vi "test spiral scan.vi"() -> ()   [LabVIEW 2010]
uses:
  scan_specification_tagResonant.ctl
panel:
  out "Waveform Chart":i16[](graph)
  out "scan pattern":cluster{i16[], i16[]}[](graph)
  out "scan specification out":T1
  out "rev scan pattern":cluster{i16[], i16[]}(graph)
  out "fwd scan pattern":cluster{i16[], i16[]}(graph)
  in  "maximum frequency":dbl=3000.0
  in  "scan specification":T1={"z resolution (pixels)"=30, "iterations per pixel"=5, "iterations per z-scan (=zres*iterperpixel)"=150, "x resolution (pixels)"=80, "y resolution (pixels)"=80, "number of z-lines per volume"=0, "number of repetitions (volumes)"=0, "Pockels cell voltage (bits)"=0, "Vx center (bits)"=0, "Vy center (bits)"=0, "Vx amplitude (bits)"=1000, "Vy amplitude (bits)"=1000, "lines to delay between scan start and output"=0, "LSB has acquire control"=FALSE}
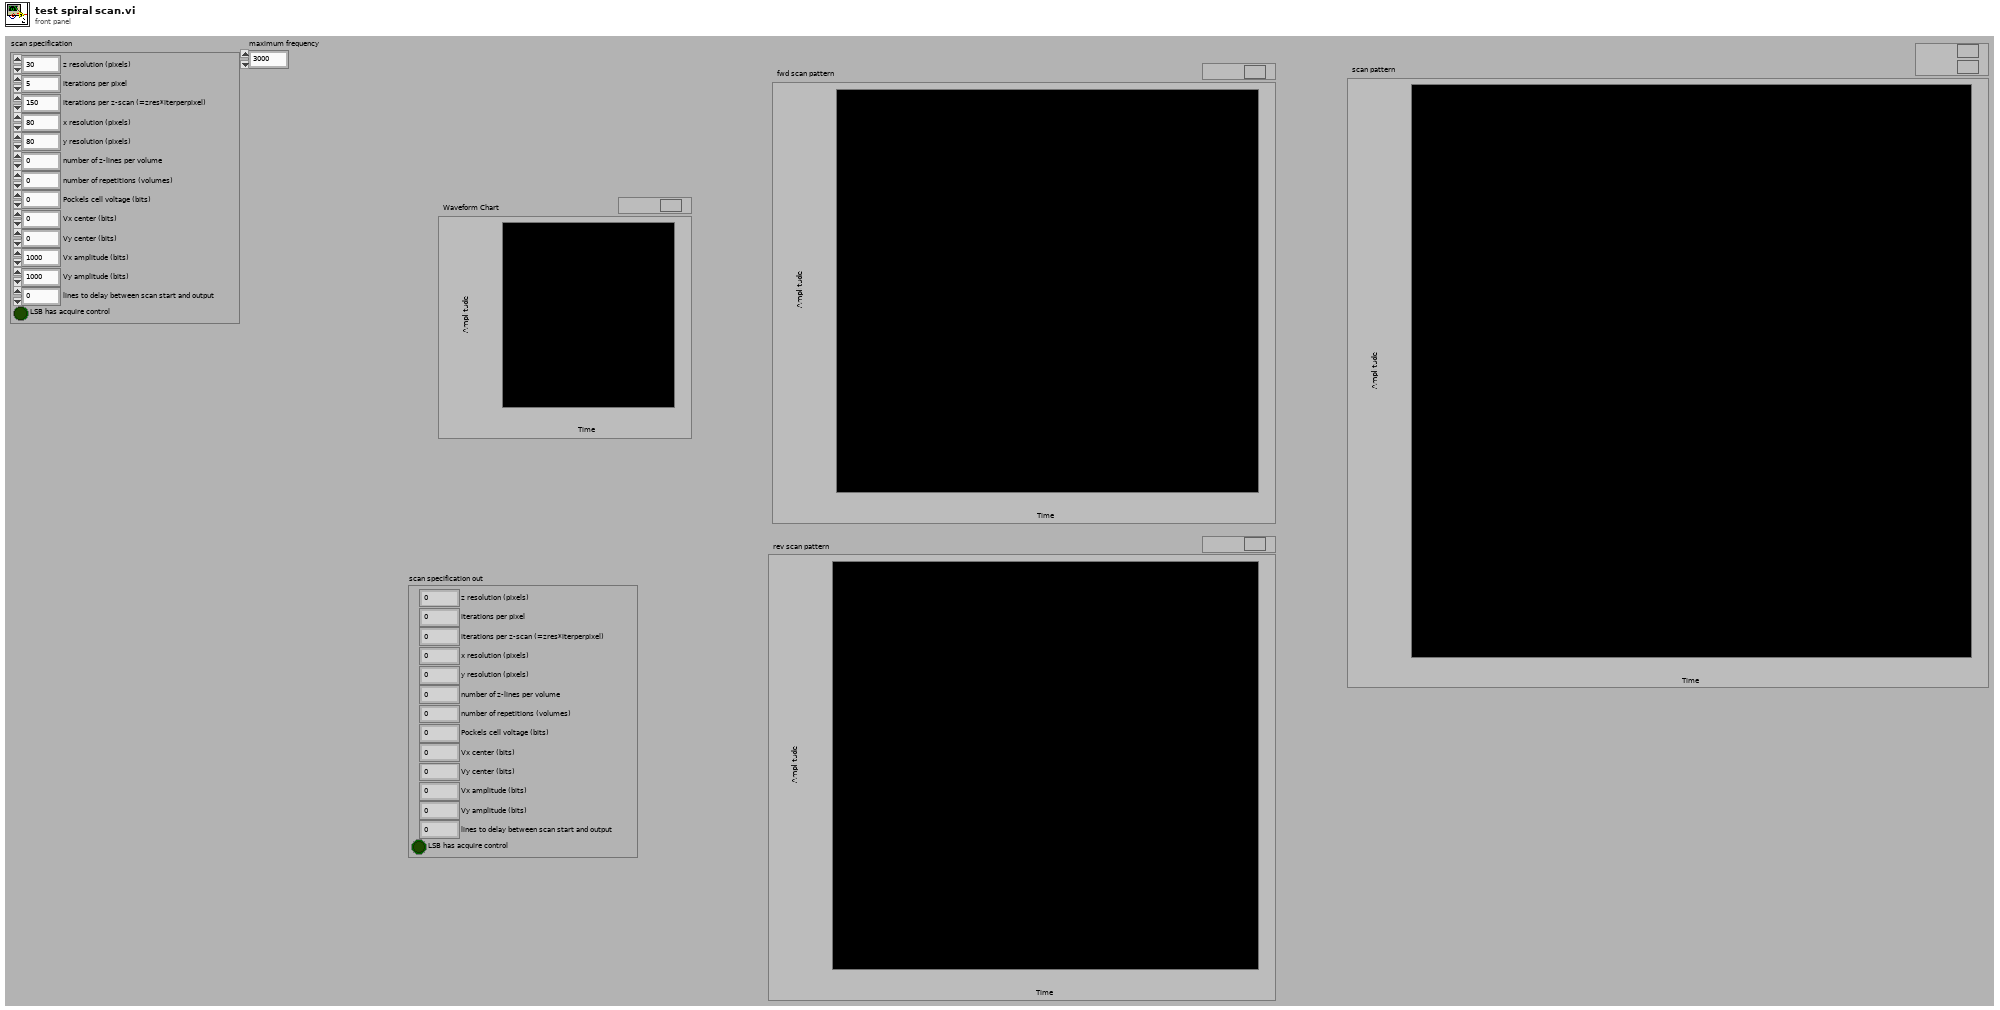
[diagram p1: front panel]
types:
  T1 = typedef "scan_specification_tagResonant.ctl" = cluster{"z resolution (pixels)":u16, "iterations per pixel":u16, "iterations per z-scan (=zres*iterperpixel)":u16, "x resolution (pixels)":u16, "y resolution (pixels)":u16, "number of z-lines per volume":u16, "number of repetitions (volumes)":i32, "Pockels cell voltage (bits)":i16, "Vx center (bits)":i16, "Vy center (bits)":i16, "Vx amplitude (bits)":i16, "Vy amplitude (bits)":i16, "lines to delay between scan start and output":u16, "LSB has acquire control":bool}
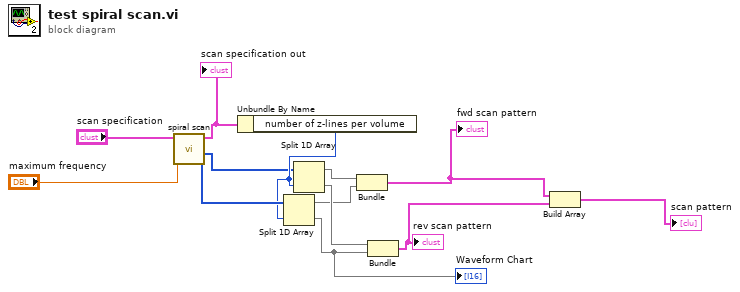
[diagram p0: block diagram]
diagram:
  n1 = call "spiral scan.vi"("maximum frequency"="maximum frequency", "scan specification"="scan specification") -> ("y"=w10:i16[], "x"=w4:i16[], "scan specification out"=w11:T1)  [unwired: 6 in, 1 out]
  "scan specification out" <- w11
  n2 = Unbundle By Name(w11) -> ("number of z-lines per volume"=w9:u16)
  n3 = Split 1D Array(array=w10, index=w9) -> (first subarray=w2:i16[], second subarray=w1:i16[])
  "Waveform Chart" <- w1
  n4 = Split 1D Array(array=w4, index=w9) -> (first subarray=w3:i16[], second subarray=w8:i16[])
  n5 = Bundle(w3, w2) -> (w7:cluster{i16[], i16[]})  [unwired: 1 in]
  "fwd scan pattern" <- w7
  n6 = Bundle(w8, w1) -> (w6:cluster{i16[], i16[]})  [unwired: 1 in]
  "rev scan pattern" <- w6
  n7 = Build Array(w7, w6) -> (→"scan pattern":cluster{i16[], i16[]}[])
